vi "SImple stream tester.vi"() -> ()   [LabVIEW 2015]
uses:
  <vilib>/visionFPGA/Controls/IMAQ FPGA Image Size.ctl
  <vilib>/FPGAPlugInAG/cRIO-9030/niLvFpga_Open_cRIO-9030.vi
  <vilib>/rvi/interface/common/dynamic/niFpgaDynamicAddResources.vi
  <vilib>/visionFPGA/Basics/Configure Image Transfer to Target/IMAQ FPGA Configure Image Transfer to Target U8.vi
  <vilib>/visionFPGA/Basics/Image Transfer to Target/IMAQ FPGA Image Transfer to Target U8.vi
  <vilib>/rvi/interface/nirviOpenFPGA/nirviOpenFPGA.xnode
  FPGA Bitfiles/BELKINEAGLE_FPGATarget_FPGAIPChainV1_CFyF0ro37YQ.lvbitx
  IP Dev Area/FPGA IP Chain V1.vi
  <vilib>/visionFPGA/NI_VDM_FPGA_Basics.lvlib
panel:
  out "error out":errorcluster
  out "Image Out":T1(plugin-control)
  out "Intensity Graph":u8[][](graph)
  out "output array":dbl[](array[numeric])
  in  "Array":u8[][](array[numeric])=[[1, 50, 100, 150], [180, 200, 230, 255]]
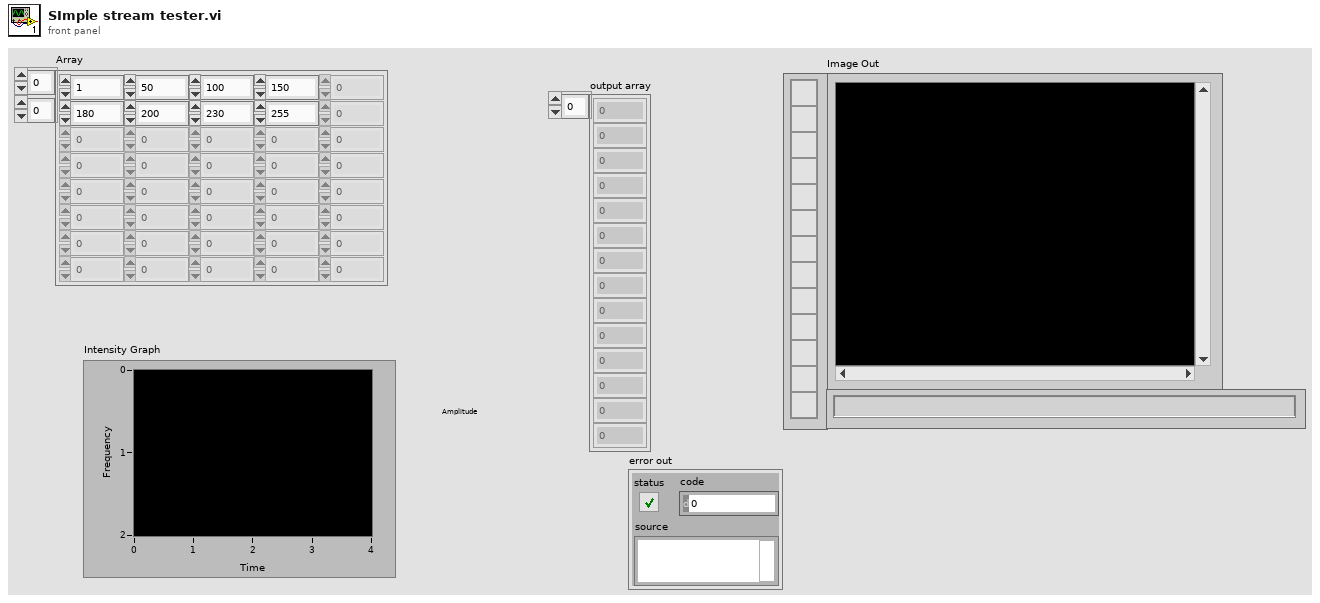
[diagram p1: front panel]
types:
  T1 = typedef "IMAQ Image.ctl" = refnum<image>
  T2 = cluster{"DMA FIFO Name":string, "Image Size Control Name":string}
  T3 = typedef "IMAQ FPGA Image Size.ctl" = cluster{"Width":u32, "Height":u32}
  T4 = typedef "Image Type" = u32
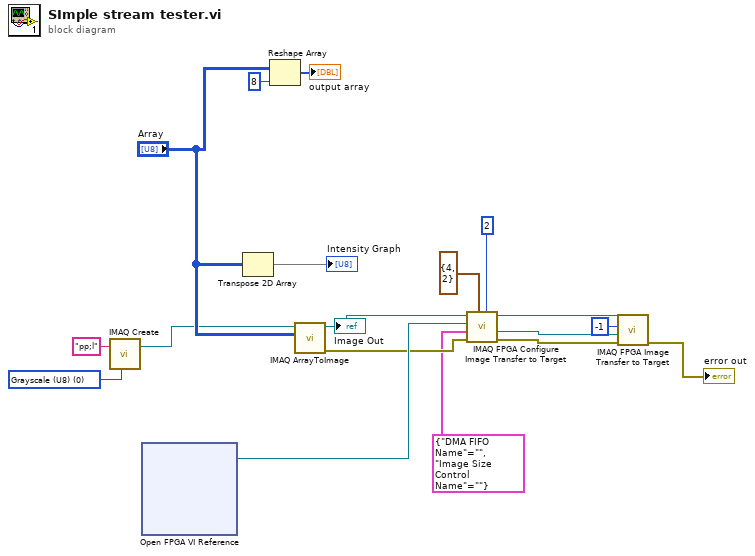
[diagram p0: block diagram]
diagram:
  w12 = T4 0 items=["Grayscale (U8)", "Grayscale (I16)", "Grayscale (SGL)", "Complex (CSG)", "RGB (U32)", "HSL (U32)", "RGB (U64)", "Grayscale (U16)"] ("Image Type")
  n1 = call "IMAQ Create"("Image Name"="pp;l", "Image Type"=w12) -> ("New Image"=w13:T1)  [unwired: 3 in, 1 out]
  n2 = xnode "Open FPGA VI Reference"() -> ("FPGA VI Reference Out"=w11:refnum<k20>)  [unwired: 2 in, 1 out]
  n3 = Transpose 2D Array(2D array="Array") -> (transposed array=→"Intensity Graph":u8[][])
  n4 = Reshape Array("Array", 8 ("dimension size")) -> (→"output array":u8[])
  n5 = call "IMAQ ArrayToImage"("Image Pixels (U8)"="Array", "Image"=w13) -> ("error out"=w10:errorcluster, "Image Out"=w2:T1)  [unwired: 8 in]
  "Image Out" <- w2
  n6 = call-poly <vilib>:"IMAQ FPGA Configure Image Transfer to Target.vi"("DMA FIFO Depth in Images"=u32 2, "Image Size"=T3 {"Width"=4, "Height"=2}, "error in (no error)"=w10, "Resource Names"=T2 {"DMA FIFO Name"="", "Image Size Control Name"=""}, "FPGA VI Reference In"=w11, "Image"=w2) -> ("error out"=w5:errorcluster, "DMA FIFO Reference Out"=w7:refnum<k20>, "Image Out"=w1:T1)  [unwired: 2 in, 1 out]
  n7 = call-poly <vilib>:"IMAQ FPGA Image Transfer to Target.vi"("error in (no error)"=w5, "DMA FIFO Reference In"=w7, "Maximum Pixels per Write"=-1, "Image"=w1) -> ("error out"=→"error out":errorcluster)  [unwired: 5 in, 2 out]
